vi "UTIL Config Analog Output.vi"(7 "Task In":refnum<k21>) -> (0 "sampling info":cluster{"Fs":dbl, "#s":dbl}, 1 "Error Out":errorcluster, 2 "Phase":dbl, 3 "Task Out":refnum<k21>)   [LabVIEW 2010]
uses:
  <vilib>/DAQmx/configure/timing.llb/DAQmx Timing (Sample Clock).vi
  Program Files (x86)/National Instruments/LabVIEW 2010/resource/objmgr/daqmx.rc
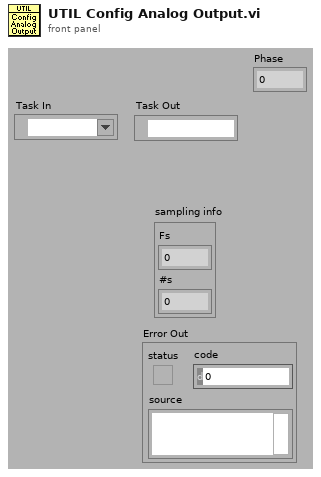
[diagram p1: front panel]
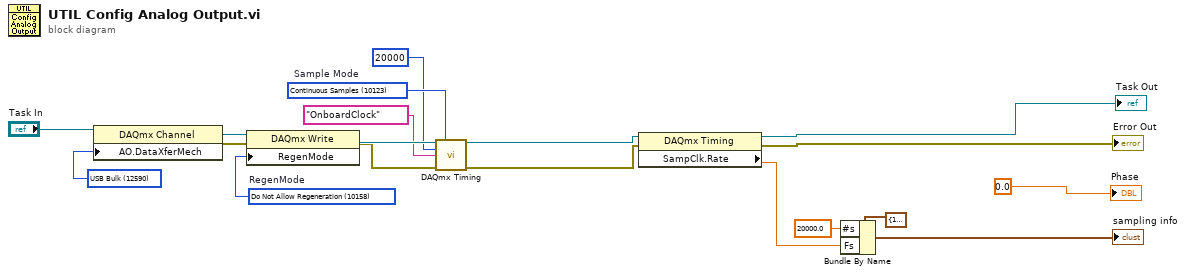
[diagram p0: block diagram]
diagram:
  w15 = 12590 items=["DMA"=10054, "Interrupts"=10204, "Programmed I/O"=10264, "USB Bulk"=12590] ("AO.DataXferMech")
  w9 = 10158 items=["Allow Regeneration"=10097, "Do Not Allow Regeneration"=10158]  # RegenMode
  w12 = 10123 items=["Finite Samples"=10178, "Continuous Samples"=10123, "Hardware Timed Single Point"=12522]  # Sample Mode
  n1 = property class="DAQmx Channel"(reference="Task In", "AO.DataXferMech"=w15) -> (reference out=w13:refnum<k21>, error out=w14:errorcluster)  [unwired: 1 in]
  n2 = property class="DAQmx Write"(reference=w13, error in=w14, "RegenMode"=w9) -> (reference out=w11:refnum<k21>, error out=w10:errorcluster)
  n3 = call-poly <vilib>:"DAQmx Timing.vi"("task/channels in"=w11, "sample mode"=w12, "rate"=20000, "source"=tag "OnboardClock" ("Sample Clock Source"), "error in"=w10) -> ("task out"=w4:refnum<k21>, "error out"=w3:errorcluster)  [unwired: 9 in]
  n4 = property class="DAQmx Timing"(reference=w4, error in=w3) -> (reference out=→"Task Out":refnum<k21>, error out=→"Error Out":errorcluster, "SampClk.Rate"=w17:dbl)
  n5 = Bundle By Name(cluster=cluster{"Fs":dbl, "#s":dbl} {"Fs"=1000.0, "#s"=1000.0} ("sampling info"), "#s"=20000.0, "Fs"=w17) -> (→"sampling info":cluster{"Fs":dbl, "#s":dbl})
  "Phase" <- 0.0 ("element")
